vi "Enviar_trama_movimiento.vi"(0 "VISA resource name":refnum<visa-resource-name>, 1 "Cluster_Tracking":T1, 5 "Tipo movimiento":T3=enum."AVANZAR", 7 "Distancia Z":T2=32000 items=["2cm"=64000, "1cm"=32000, "1mm"=3200, "0.5mm"=1600], 9 "Distancia X/Y":T4 items=["10cm"=9100, "1cm"=910, "1mm"=91, "0.1mm"=9, "1 paso "=1], 11 "error in (no error)":errorcluster) -> (4 "VISA resource name 2":refnum<visa-resource-name>, 6 "TRAMA ENVIADA":string, 10 "Tipo movimiento":T3=enum."AVANZAR", 15 "error out":errorcluster)   [LabVIEW 2019]
uses:
  Typedefs/Tipo_movimiento.ctl
  Typedefs/Distancia.ctl
  Typedefs/Distancia_Z.ctl
  Typedefs/Cluster_tracking.ctl
  <vilib>/Utility/error.llb/Error Cluster From Error Code.vi
  <vilib>/ErrorRing/Error Ring.xnode
panel:
  out "Cluster_Tracking 2":T1
  out "TRAMA ENVIADA CORRECTAMENTE?":bool
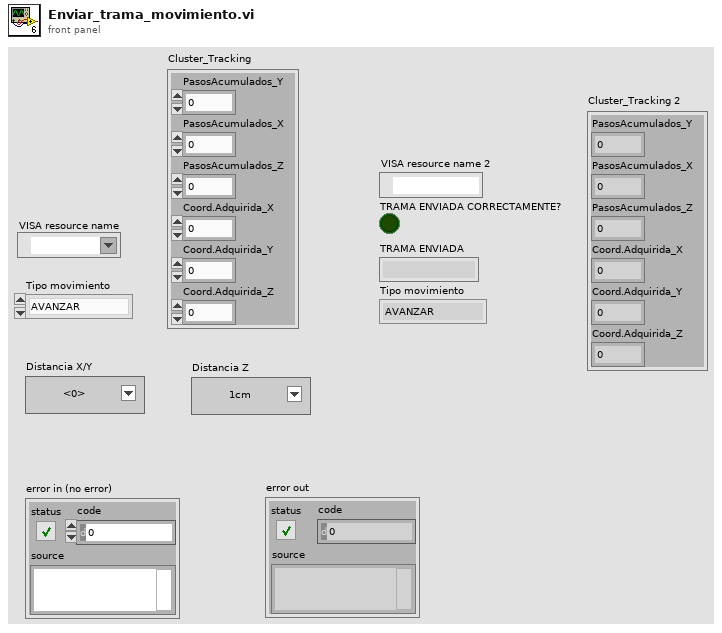
[diagram p1: front panel]
types:
  T1 = typedef "Cluster_tracking.ctl" = cluster{"PasosAcumulados_Y":i32, "PasosAcumulados_X":i32, "PasosAcumulados_Z":i32, "Coord.Adquirida_X":i32, "Coord.Adquirida_Y":i32, "Coord.Adquirida_Z":i32}
  T2 = typedef "Distancia_Z.ctl" = i32
  T3 = typedef "Tipo_movimiento.ctl" = enum16{"NINGUNO", "AVANZAR", "RETROCEDER", "DERECHA", "IZQUIERDA", "SUBIRZ", "BAJARZ", "HOME", "HOME_Z"}
  T4 = typedef "Distancia.ctl" = i32
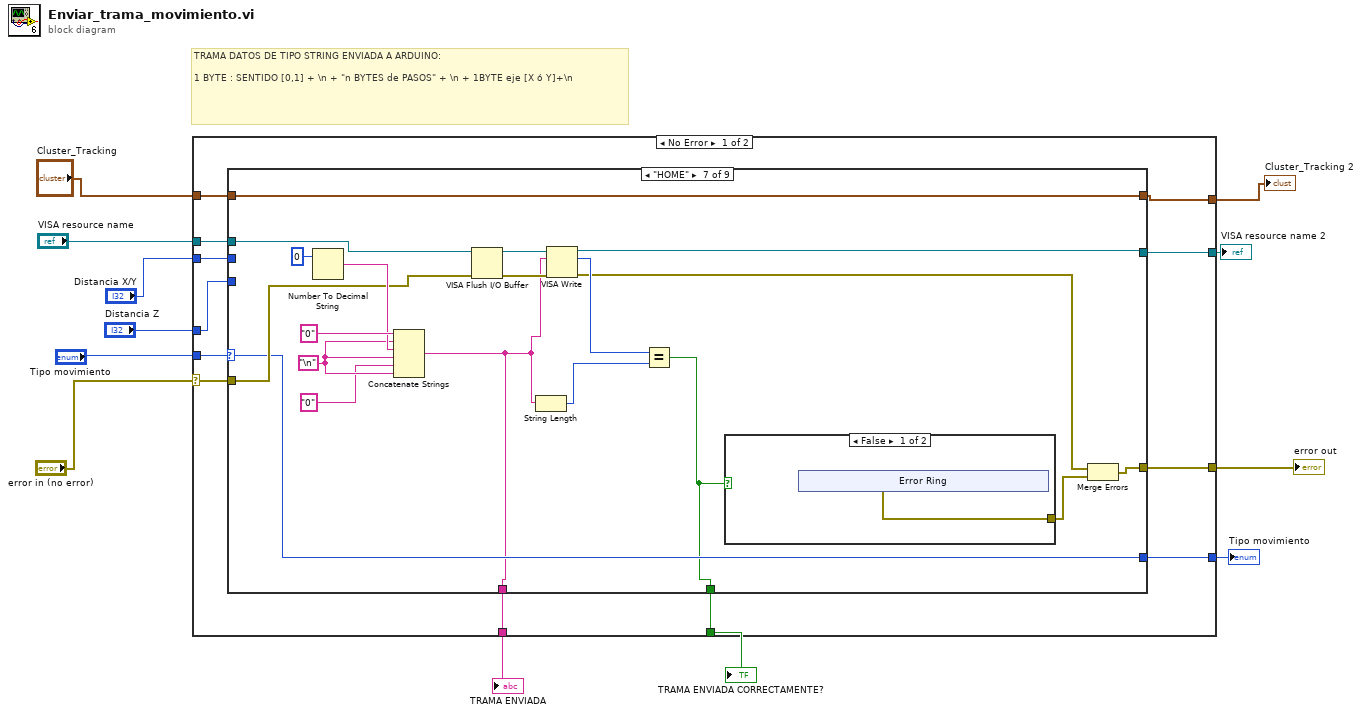
[diagram p0: block diagram]
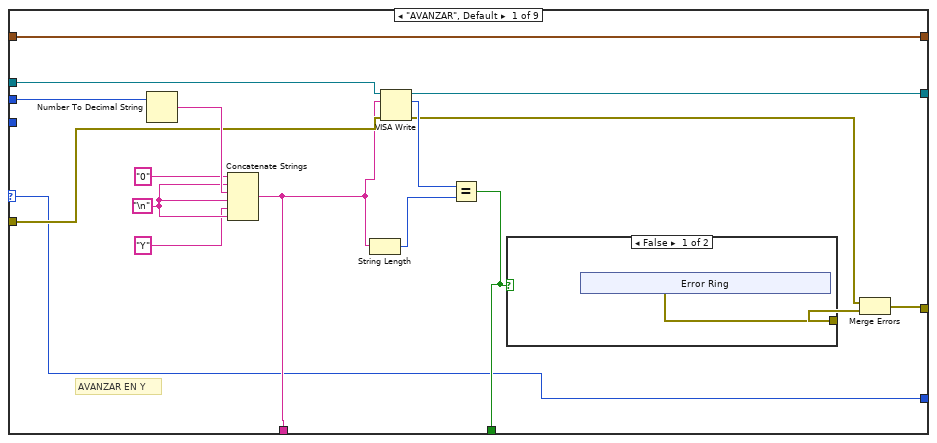
[diagram p2: hidden frame]
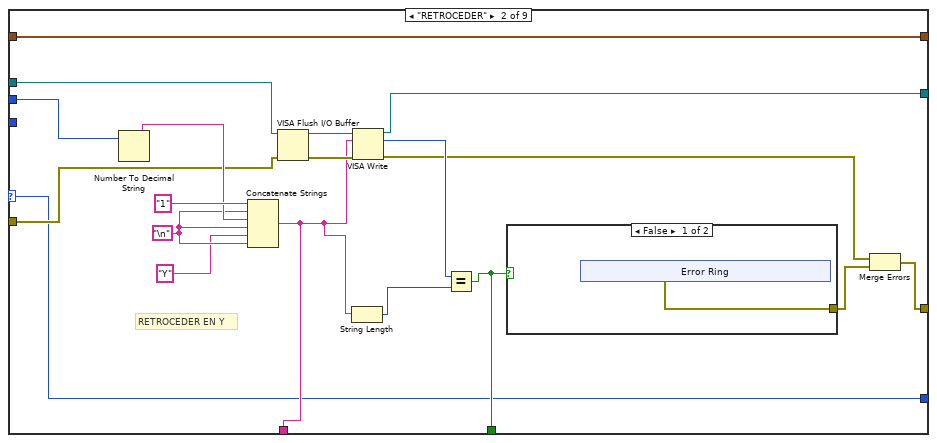
[diagram p4: hidden frame]
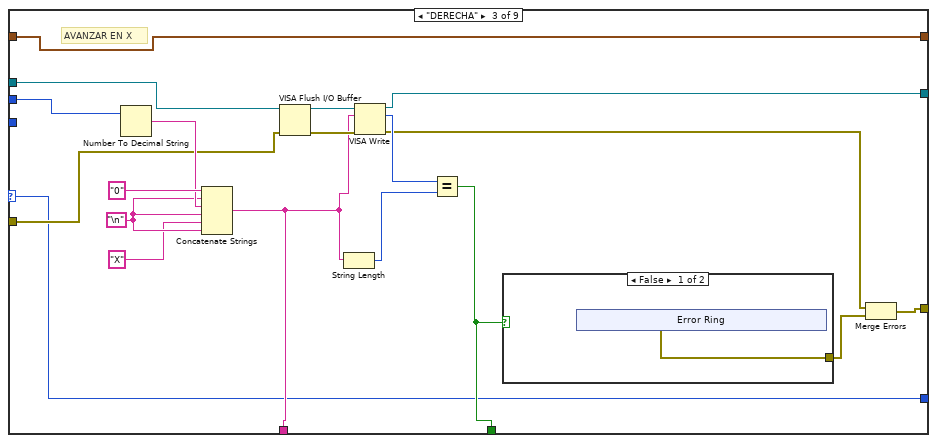
[diagram p6: hidden frame]
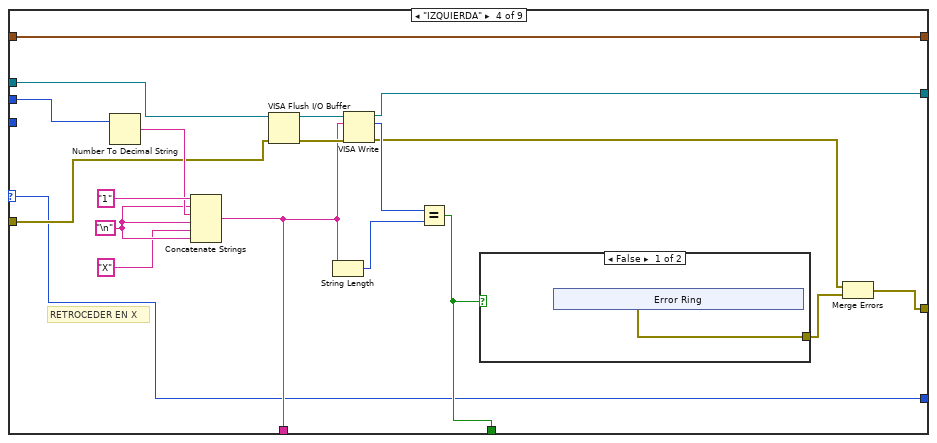
[diagram p8: hidden frame]
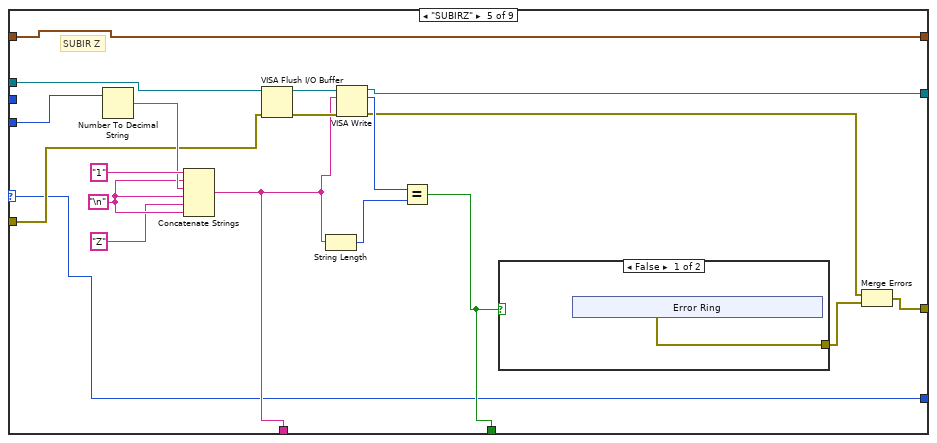
[diagram p10: hidden frame]
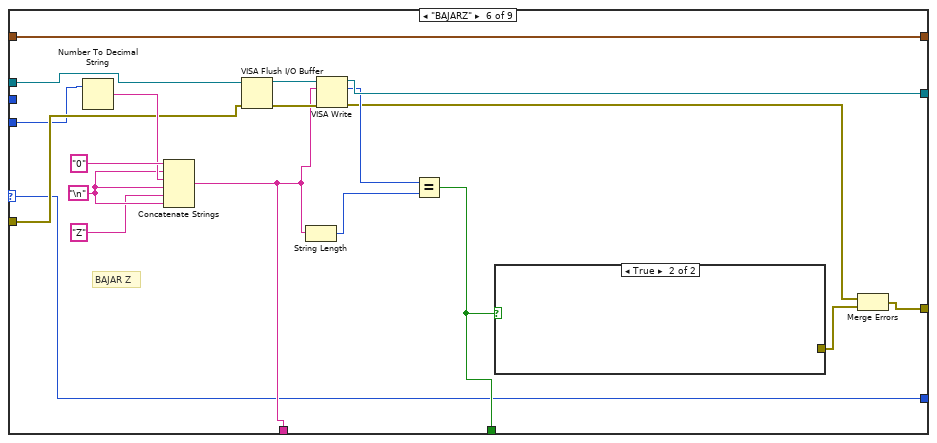
[diagram p12: hidden frame]
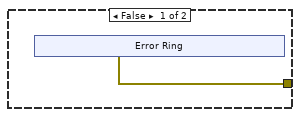
[diagram p13: hidden frame]
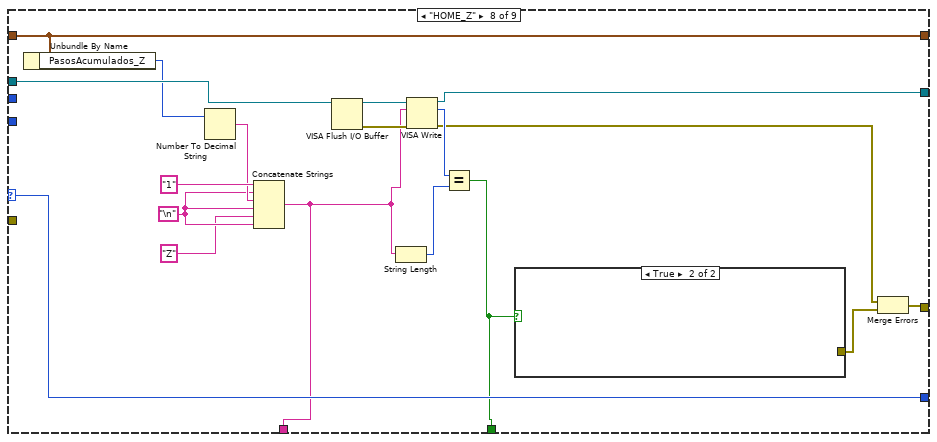
[diagram p15: hidden frame]
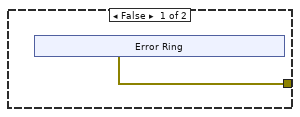
[diagram p16: hidden frame]
diagram:
  # "TRAMA DATOS DE TIPO STRING ENVIADA A ARDUINO:\n\n1 BYTE : SENTIDO [0,1] + \\n + \"n BYTES de PASOS\" + \\n + 1BYTE eje [X ó Y]+\\n"
  n1 = case shown="No Error" "error in (no error)" {
    selector: "error in (no error)" -> [w20 w229]
    tunnel: "Tipo movimiento" -> [w24 w227]
    tunnel: "Distancia X/Y" -> [w23 _]
    tunnel: [w19 w229] -> w9
    tunnel: "VISA resource name" -> [w22 w228]
    tunnel: [w21 w228] -> w7
    tunnel: [w18 _] -> w6
    tunnel: [w17 _] -> w5
    tunnel: [w16 w227] -> w4
    tunnel: "Distancia Z" -> [w15 _]
    tunnel: "Cluster_Tracking" -> [w14 w226]
    tunnel: [w13 w226] -> w1
    frame No Error {
      n2 = case shown="\"HOME\"" w24 {
        selector: w24 -> [w26 w49 w74 w99 w125 w150 w176 w204 w224]
        tunnel: w23 -> [w37 w60 w85 w107 _ _ _ _ _]
        tunnel: w22 -> [w36 w59 w84 w110 w135 w160 w180 w205 w225]
        tunnel: [w35 w58 w82 w108 w134 w158 w179 w201 w225] -> w21
        tunnel: w20 -> [w34 w57 w83 w109 w133 w159 w177 _ w223]
        tunnel: [w29 w52 w77 w102 w127 w153 w178 w203 w223] -> w19
        tunnel: [w28 w51 w76 w101 w132 w152 w175 w198 _] -> w18
        tunnel: [w27 w50 w75 w100 w126 w151 w174 w199 _] -> w17
        tunnel: [w26 w49 w74 w99 w125 w150 w176 w204 w224] -> w16
        tunnel: w15 -> [_ _ _ _ w124 w149 _ _ _]
        tunnel: w14 -> [w25 w48 w73 w98 w123 w148 w173 w200 w222]
        tunnel: [w25 w48 w73 w98 w123 w148 w173 w200 w222] -> w13
        frame "AVANZAR", Default {
          w39 = "\n"
          # "AVANZAR EN Y"
          n3 = Number To Decimal String(number=w37) -> (decimal integer string=w41:string)  [unwired: 1 in]
          n4 = Concatenate Strings("0", w39, w41, w39, "Y" ("string"), w39) -> (w28:string)
          n5 = String Length(string=w28) -> (length=w32:i32)
          n6 = VISA Write(VISA resource name=w36, write buffer=w28, error in (no error)=w34) -> (VISA resource name out=w35:refnum<visa-resource-name>, return count=w31:u32, error out=w30:errorcluster)
          n7 = Equal?(x=w31, y=w32) -> (x = y?=w27:bool)
          n8 = case shown="False" w27 {
            tunnel: [w42 _] -> w33
            frame False {
              n9 = xnode "Error Ring"() -> ("error out"=w42:errorcluster)
            }
            frame True {
            }
          }
          n10 = Merge Errors(w30, w33) -> (w29:errorcluster)
        }
        frame "RETROCEDER" {
          w62 = "\n"
          # "RETROCEDER EN Y"
          n11 = Number To Decimal String(number=w60) -> (decimal integer string=w63:string)  [unwired: 1 in]
          n12 = Concatenate Strings("1", w62, w63, w62, "Y" ("string"), w62) -> (w51:string)
          n13 = VISA Flush I/O Buffer(VISA resource name=w59, error in (no error)=w57) -> (VISA resource name out=w65:refnum<visa-resource-name>, error out=w66:errorcluster)  [unwired: 1 in]
          n14 = String Length(string=w51) -> (length=w55:i32)
          n15 = VISA Write(VISA resource name=w65, write buffer=w51, error in (no error)=w66) -> (VISA resource name out=w58:refnum<visa-resource-name>, return count=w56:u32, error out=w54:errorcluster)
          n16 = Equal?(x=w56, y=w55) -> (x = y?=w50:bool)
          n17 = case shown="False" w50 {
            tunnel: [w67 _] -> w53
            frame False {
              n18 = xnode "Error Ring"() -> ("error out"=w67:errorcluster)
            }
            frame True {
            }
          }
          n19 = Merge Errors(w54, w53) -> (w52:errorcluster)
        }
        frame "DERECHA" {
          w87 = "\n"
          # "AVANZAR EN X"
          n20 = Number To Decimal String(number=w85) -> (decimal integer string=w88:string)  [unwired: 1 in]
          n21 = Concatenate Strings("0", w87, w88, w87, "X" ("string"), w87) -> (w76:string)
          n22 = VISA Flush I/O Buffer(VISA resource name=w84, error in (no error)=w83) -> (VISA resource name out=w90:refnum<visa-resource-name>, error out=w91:errorcluster)  [unwired: 1 in]
          n23 = String Length(string=w76) -> (length=w79:i32)
          n24 = VISA Write(VISA resource name=w90, write buffer=w76, error in (no error)=w91) -> (VISA resource name out=w82:refnum<visa-resource-name>, return count=w80:u32, error out=w78:errorcluster)
          n25 = Equal?(x=w80, y=w79) -> (x = y?=w75:bool)
          n26 = case shown="False" w75 {
            tunnel: [w92 _] -> w81
            frame False {
              n27 = xnode "Error Ring"() -> ("error out"=w92:errorcluster)
            }
            frame True {
            }
          }
          n28 = Merge Errors(w78, w81) -> (w77:errorcluster)
        }
        frame "IZQUIERDA" {
          w112 = "\n"
          # "RETROCEDER EN X"
          n29 = Number To Decimal String(number=w107) -> (decimal integer string=w113:string)  [unwired: 1 in]
          n30 = Concatenate Strings("1", w112, w113, w112, "X" ("string"), w112) -> (w101:string)
          n31 = VISA Flush I/O Buffer(VISA resource name=w110, error in (no error)=w109) -> (VISA resource name out=w115:refnum<visa-resource-name>, error out=w116:errorcluster)  [unwired: 1 in]
          n32 = String Length(string=w101) -> (length=w105:i32)
          n33 = VISA Write(VISA resource name=w115, write buffer=w101, error in (no error)=w116) -> (VISA resource name out=w108:refnum<visa-resource-name>, return count=w104:u32, error out=w103:errorcluster)
          n34 = Equal?(x=w104, y=w105) -> (x = y?=w100:bool)
          n35 = case shown="False" w100 {
            tunnel: [w117 _] -> w106
            frame False {
              n36 = xnode "Error Ring"() -> ("error out"=w117:errorcluster)
            }
            frame True {
            }
          }
          n37 = Merge Errors(w103, w106) -> (w102:errorcluster)
        }
        frame "SUBIRZ" {
          w137 = "\n"
          # "SUBIR Z"
          n38 = Number To Decimal String(number=w124) -> (decimal integer string=w138:string)  [unwired: 1 in]
          n39 = Concatenate Strings("1", w137, w138, w137, "Z" ("string"), w137) -> (w132:string)
          n40 = VISA Flush I/O Buffer(VISA resource name=w135, error in (no error)=w133) -> (VISA resource name out=w140:refnum<visa-resource-name>, error out=w141:errorcluster)  [unwired: 1 in]
          n41 = String Length(string=w132) -> (length=w130:i32)
          n42 = VISA Write(VISA resource name=w140, write buffer=w132, error in (no error)=w141) -> (VISA resource name out=w134:refnum<visa-resource-name>, return count=w129:u32, error out=w128:errorcluster)
          n43 = Equal?(x=w129, y=w130) -> (x = y?=w126:bool)
          n44 = case shown="False" w126 {
            tunnel: [w142 _] -> w131
            frame False {
              n45 = xnode "Error Ring"() -> ("error out"=w142:errorcluster)
            }
            frame True {
            }
          }
          n46 = Merge Errors(w128, w131) -> (w127:errorcluster)
        }
        frame "BAJARZ" {
          w162 = "\n"
          # "BAJAR Z"
          n47 = Number To Decimal String(number=w149) -> (decimal integer string=w163:string)  [unwired: 1 in]
          n48 = Concatenate Strings("0", w162, w163, w162, "Z" ("string"), w162) -> (w152:string)
          n49 = VISA Flush I/O Buffer(VISA resource name=w160, error in (no error)=w159) -> (VISA resource name out=w165:refnum<visa-resource-name>, error out=w166:errorcluster)  [unwired: 1 in]
          n50 = String Length(string=w152) -> (length=w156:i32)
          n51 = VISA Write(VISA resource name=w165, write buffer=w152, error in (no error)=w166) -> (VISA resource name out=w158:refnum<visa-resource-name>, return count=w155:u32, error out=w154:errorcluster)
          n52 = Equal?(x=w155, y=w156) -> (x = y?=w151:bool)
          n53 = case shown="True" w151 {
            tunnel: [w167 _] -> w157
            frame False {
              n54 = xnode "Error Ring"() -> ("error out"=w167:errorcluster)
            }
            frame True {
            }
          }
          n55 = Merge Errors(w154, w157) -> (w153:errorcluster)
        }
        frame "HOME" {
          w187 = "\n"
          n56 = Number To Decimal String(number=0) -> (decimal integer string=w188:string)  [unwired: 1 in]
          n57 = Concatenate Strings("0", w187, w188, w187, "0" ("string"), w187) -> (w175:string)
          n58 = VISA Flush I/O Buffer(VISA resource name=w180, error in (no error)=w177) -> (VISA resource name out=w190:refnum<visa-resource-name>, error out=w191:errorcluster)  [unwired: 1 in]
          n59 = String Length(string=w175) -> (length=w184:i32)
          n60 = VISA Write(VISA resource name=w190, write buffer=w175, error in (no error)=w191) -> (VISA resource name out=w179:refnum<visa-resource-name>, return count=w183:u32, error out=w182:errorcluster)
          n61 = Equal?(x=w183, y=w184) -> (x = y?=w174:bool)
          n62 = case shown="False" w174 {
            tunnel: [w192 _] -> w185
            frame False {
              n63 = xnode "Error Ring"() -> ("error out"=w192:errorcluster)
            }
            frame True {
            }
          }
          n64 = Merge Errors(w182, w185) -> (w178:errorcluster)
        }
        frame "HOME_Z" {
          w211 = "\n"
          n65 = Unbundle By Name(w200) -> ("PasosAcumulados_Z"=w202:i32)
          n66 = Number To Decimal String(number=w202) -> (decimal integer string=w212:string)  [unwired: 1 in]
          n67 = Concatenate Strings("1", w211, w212, w211, "Z" ("string"), w211) -> (w198:string)
          n68 = VISA Flush I/O Buffer(VISA resource name=w205) -> (VISA resource name out=w214:refnum<visa-resource-name>, error out=w215:errorcluster)  [unwired: 2 in]
          n69 = String Length(string=w198) -> (length=w207:i32)
          n70 = VISA Write(VISA resource name=w214, write buffer=w198, error in (no error)=w215) -> (VISA resource name out=w201:refnum<visa-resource-name>, return count=w208:u32, error out=w206:errorcluster)
          n71 = Equal?(x=w208, y=w207) -> (x = y?=w199:bool)
          n72 = case shown="True" w199 {
            tunnel: [w216 _] -> w209
            frame False {
              n73 = xnode "Error Ring"() -> ("error out"=w216:errorcluster)
            }
            frame True {
            }
          }
          n74 = Merge Errors(w206, w209) -> (w203:errorcluster)
        }
        frame "NINGUNO" {
        }
      }
    }
    frame Error {
    }
  }
  "error out" <- w9
  "VISA resource name 2" <- w7
  "TRAMA ENVIADA" <- w6
  "TRAMA ENVIADA CORRECTAMENTE?" <- w5
  "Tipo movimiento" <- w4
  "Cluster_Tracking 2" <- w1
